vi "ToplevelProbeStationControl.vi"() -> ()   [LabVIEW 2014]
uses:
  c_InstructionEnum.ctl
  g_Stop.vi
  g_CommandParam.vi
  g_ECS02_Command.vi
panel:
  in  "Stop":bool
  out "Image 2":T1(plugin-control)
  in  "Interface Name":string="img0"
  out "Y 2":dbl
  out "X 2":dbl
  in  "Calibrate":bool
  in  "COM Port MicroZed":refnum<visa-resource-name>="COM4"
  in  "StateMachineClosed":bool=TRUE
  in  "Start":bool
  in  "Y Steps":dbl
  in  "X Steps":dbl=1.0
  in  "Plate Position":i32(listbox)=1
  in  "Command":i32(listbox)=2
  in  "Y":dbl
  in  "X":dbl
  in  "X Stepsize":dbl=0.01
  in  "Y Stepsize":dbl=0.01
  in  "Load":bool
  in  "Home":bool
  in  "COM Port ECS02":refnum<visa-resource-name>="COM3"
  in  "stop":bool
  out "Write":bool
  in  "Send":bool
  # "Manual Probe Station Control"
  # "Absolute Movements"
  # "Increment"
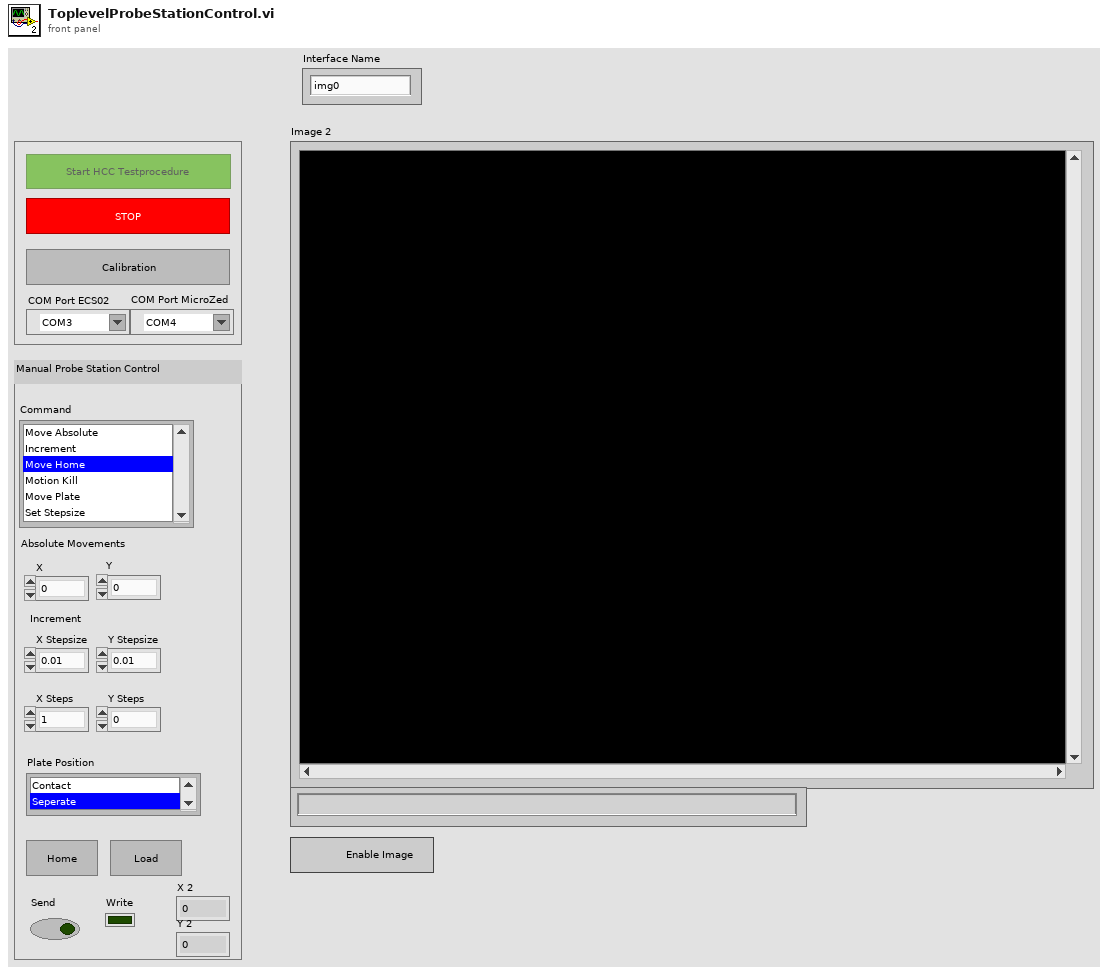
[diagram p1: front panel]
types:
  T1 = typedef "IMAQ Image.ctl" = refnum<image>
  T2 = typedef "c_InstructionEnum.ctl" = enum16{"Move Absolute", "Increment", "Move Home", "Motion Kill", "Move Plate", "Set Stepsize", "Query Position"}
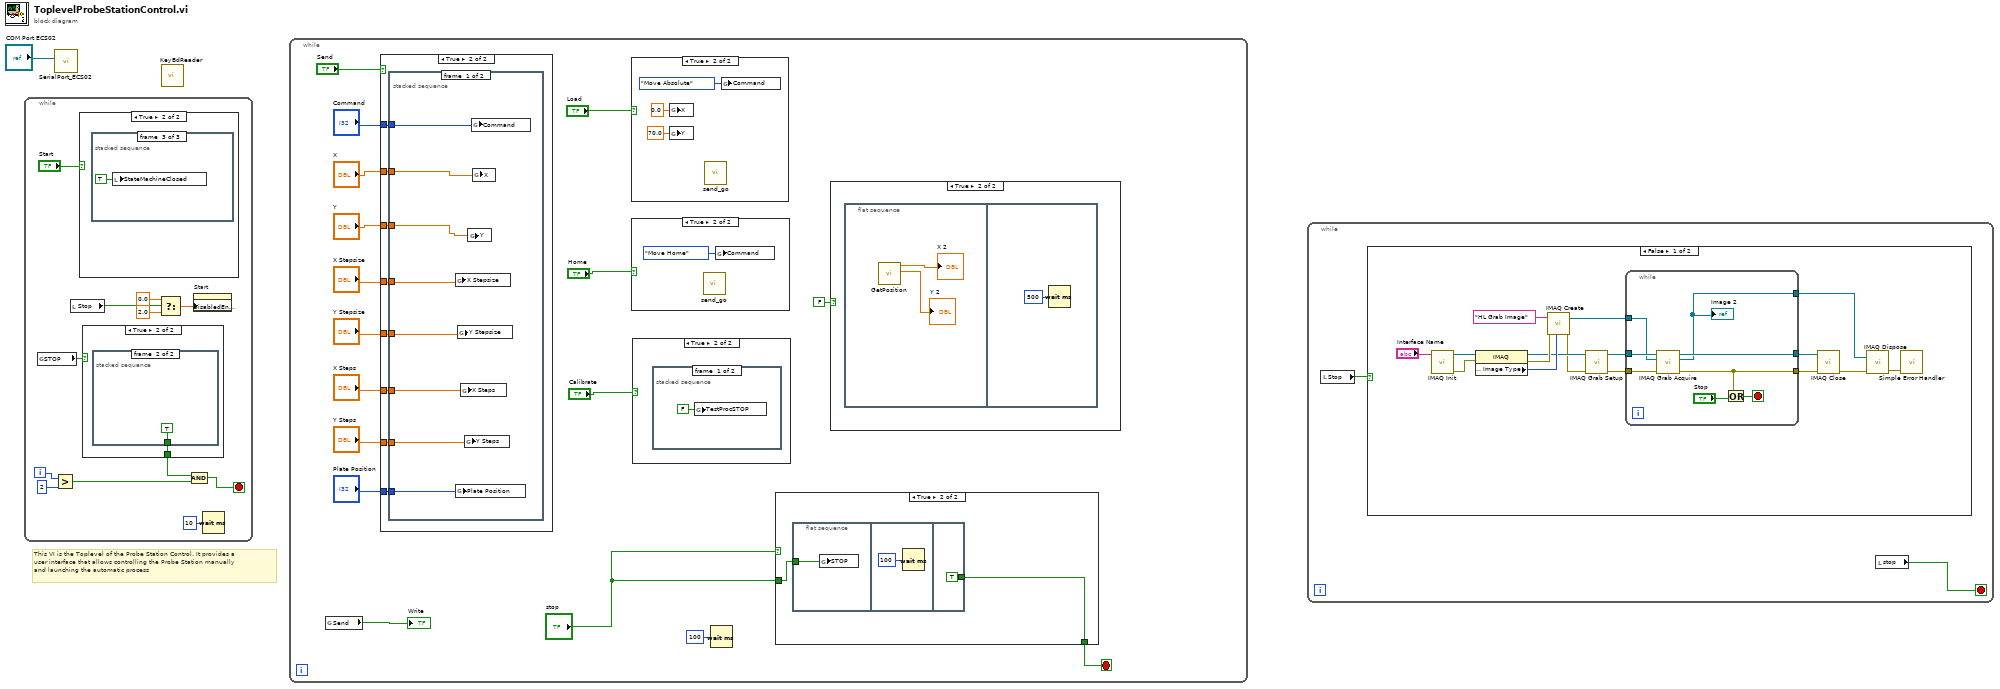
[diagram p0: block diagram]
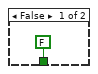
[diagram p3: hidden frame]
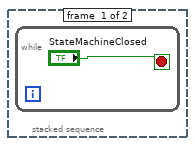
[diagram p4: hidden frame]
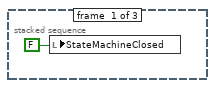
[diagram p6: hidden frame]
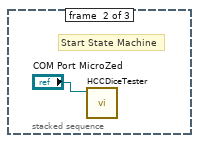
[diagram p7: hidden frame]
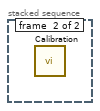
[diagram p10: hidden frame]
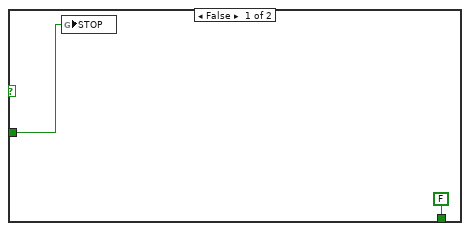
[diagram p13: hidden frame]
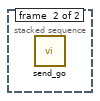
[diagram p15: hidden frame]
diagram:
  # "This VI is the Toplevel of the Probe Station Control. It provides a \nuser interface that allows controlling the Probe Station manually\nand launching the automatic process"
  n1 = while {
    i -> [w7]
    stop <- w12 stop-if-true
    n2 = global read "g_Stop.vi" "STOP"() -> (w10:bool)
    n3 = Greater?(x=w7, y=2 ("x")) -> (0:w11:bool)
    n4 = local read "Stop"() -> (w4:bool)
    n5 = case shown="True" "Start" {
      frame False {
      }
      frame True {
        n6 = stacked-sequence {
          frame #0 {
            n7 = local write "StateMachineClosed"(FALSE) -> ()
          }
          frame #1 {
            # "Start State Machine"
            n8 = call "HCCDiceTester.vi"("COM Port MicroZed"="COM Port MicroZed") -> ()  [unwired: 11 in]
          }
          frame #2 {
            n9 = local write "StateMachineClosed"(TRUE ("StateMachineClosed")) -> ()
          }
        }
      }
    }
    n10 = case shown="True" w10 {
      tunnel: [FALSE w15] -> w9
      frame False {
      }
      frame True {
        n11 = stacked-sequence {
          tunnel: [_ TRUE] -> w15
          frame #0 {
            n12 = while {
              stop <- "StateMachineClosed" stop-if-true
            }
          }
          frame #1 {
          }
        }
      }
    }
    n13 = Select(t=0.0, s=w4, f=2.0) -> (s? t:f=w5:dbl)
    n14 = Compound Arithmetic op=AND(w9, w11) -> (w12:bool)
    n15 = property on="Start" class="Bool"("DisabledEnum"=w5) -> ()  [unwired: 2 in, 2 out]
    n16 = Wait (ms)(milliseconds to wait=u32 10) -> ()  [unwired: 1 out]
  }
  n17 = call "SerialPort_ECS02.vi"("COM Port"="COM Port ECS02") -> ()  [unwired: 2 in, 1 out]
  n18 = call "KeyBdReader.vi"() -> ()  [unwired: 11 in, 1 out]
  n19 = while {
    stop <- w24 stop-if-true
    n20 = global read "g_ECS02_Command.vi" "Send"() -> (→"Write":bool)
    n21 = case shown="True" "Send" {
      tunnel: "Command" -> [_ w60]
      tunnel: "X" -> [_ w59]
      tunnel: "Y" -> [_ w58]
      tunnel: "X Stepsize" -> [_ w57]
      tunnel: "Y Stepsize" -> [_ w56]
      tunnel: "X Steps" -> [_ w55]
      tunnel: "Y Steps" -> [_ w54]
      tunnel: "Plate Position" -> [_ w53]
      frame False {
      }
      frame True {
        n22 = stacked-sequence {
          tunnel: w60 -> [w68 _]
          tunnel: w59 -> [w67 _]
          tunnel: w58 -> [w66 _]
          tunnel: w57 -> [w65 _]
          tunnel: w56 -> [w64 _]
          tunnel: w55 -> [w63 _]
          tunnel: w54 -> [w62 _]
          tunnel: w53 -> [w61 _]
          frame #0 {
            n23 = global write "g_CommandParam.vi" "X Stepsize"(w65) -> ()
            n24 = global write "g_CommandParam.vi" "Plate Position"(w61) -> ()
            n25 = global write "g_CommandParam.vi" "Y Stepsize"(w64) -> ()
            n26 = global write "g_CommandParam.vi" "X Steps"(w63) -> ()
            n27 = global write "g_CommandParam.vi" "Y Steps"(w62) -> ()
            n28 = global write "g_CommandParam.vi" "Y"(w66) -> ()
            n29 = global write "g_CommandParam.vi" "Command"(w68) -> ()
            n30 = global write "g_CommandParam.vi" "X"(w67) -> ()
          }
          frame #1 {
            n31 = call "send_go.vi"() -> ()  [unwired: 12 in]
          }
        }
      }
    }
    n32 = case shown="True" "Load" {
      frame False {
      }
      frame True {
        n33 = global write "g_CommandParam.vi" "X"(0.0 ("X")) -> ()
        n34 = global write "g_CommandParam.vi" "Y"(70.0 ("X")) -> ()
        n35 = call "send_go.vi"() -> ()  [unwired: 12 in]
        n36 = global write "g_CommandParam.vi" "Command"(c_InstructionEnum."Move Absolute" ("Command")) -> ()
      }
    }
    n37 = case shown="True" "Home" {
      frame False {
      }
      frame True {
        n38 = call "send_go.vi"() -> ()  [unwired: 12 in]
        n39 = global write "g_CommandParam.vi" "Command"(c_InstructionEnum."Move Home" ("Command")) -> ()
      }
    }
    n40 = case shown="True" "Calibrate" {
      frame False {
      }
      frame True {
        n41 = stacked-sequence {
          frame #0 {
            n42 = global write "g_Stop.vi" "TestProcSTOP"(FALSE ("TestProcSTOP")) -> ()
          }
          frame #1 {
            n43 = call "Calibration.vi"() -> ()  [unwired: 12 in]
          }
        }
      }
    }
    n44 = Wait (ms)(milliseconds to wait=u32 100) -> ()  [unwired: 1 out]
    n45 = case shown="True" "stop" {
      tunnel: "stop" -> [w47 w49]
      tunnel: [FALSE w48] -> w24
      frame False {
        n46 = global write "g_Stop.vi" "STOP"(w47) -> ()
      }
      frame True {
        n47 = flat-sequence {
          tunnel: w49 -> [w50]
          tunnel: [TRUE] -> w48
          frame #0 {
            n48 = global write "g_Stop.vi" "STOP"(w50) -> ()
          }
          frame #1 {
            n49 = Wait (ms)(milliseconds to wait=u32 100) -> ()  [unwired: 1 out]
          }
          frame #2 {
          }
        }
      }
    }
    n50 = case shown="True" FALSE {
      frame False {
      }
      frame True {
        n51 = flat-sequence {
          frame #0 {
            n52 = call "GetPosition.vi"() -> ("Y"=→"Y 2":dbl, "X"=→"X 2":dbl)  [unwired: 10 in]
          }
          frame #1 {
            n53 = Wait (ms)(milliseconds to wait=u32 500) -> ()  [unwired: 1 out]
          }
        }
      }
    }
  }
  n54 = while {
    stop <- w70 stop-if-true
    n55 = local read "Stop"() -> (w69:bool)
    n56 = case shown="False" w69 {
      frame False {
        n57 = call <vilib>:"IMAQ Init.vi"("Interface Name"="Interface Name") -> ("error out"=w79:errorcluster, "IMAQ Session Out"=w78:refnum<k11>)  [unwired: 1 in, 8 out]
        n58 = property class="IMAQ"(reference=w78, error in=w79) -> (reference out=w80:refnum<k11>, error out=w81:errorcluster, "Image Parameters : Image Type"=w82:u32)
        n59 = call "IMAQ Create"("Image Name"="HL Grab Image", "Image Type"=w82, "error in (no error)"=w81) -> ("New Image"=w72:T1, "error out"=w71:errorcluster)  [unwired: 1 in, 1 out]
        n60 = call <vilib>:"IMAQ Grab Setup.vi"("error in (no error)"=w71, "IMAQ Session In"=w80) -> ("error out"=w74:errorcluster, "IMAQ Session Out"=w73:refnum<k11>)  [unwired: 8 out]
        n61 = while {
          tunnel: [w89] -> w77
          tunnel: w72 -> [w92]
          tunnel: w73 -> [w93]
          tunnel: w74 -> [w94]
          tunnel: [w87] -> w83
          tunnel: [w88] -> w85
          stop <- w91 stop-if-true
          n62 = call <vilib>:"IMAQ Grab Acquire.vi"("error in (no error)"=w94, "Image In"=w92, "IMAQ Session In"=w93) -> ("error out"=w87:errorcluster, "Image Out"=w88:T1, "IMAQ Session Out"=w89:refnum<k11>)  [unwired: 1 in, 5 out]
          "Image 2" <- w88
          n63 = Or(x=w87, y="Stop") -> (x .or. y?=w91:bool)
        }
        n64 = call <vilib>:"IMAQ Close.vi"("error in (no error)"=w83, "IMAQ Session In"=w77) -> ("error out"=w84:errorcluster)  [unwired: 9 out]
        n65 = call "IMAQ Dispose"("Image"=w85, "error in (no error)"=w84) -> ("error out"=w86:errorcluster)  [unwired: 1 in, 3 out]
        n66 = call <vilib>:"Simple Error Handler.vi"("error in (no error)"=w86) -> ()  [unwired: 1 in, 8 out]
      }
      frame True {
      }
    }
    n67 = local read "stop"() -> (w70:bool)
  }
